vi "niRFUtil FTW Apply Window (complex wfm).vi"(3 "Window":T1=enum."Gaussian", 5 "Waveform In":T2 {"y" format="%.2f"; "dx" format="%^.2e"; "x0" format="%^.2e"}) -> (0 "-ENBW (dB-Hz)":sgl format="%.2f", 1 "Coherent Loss (dB)":sgl format="%.2f", 2 "Waveform Out":T2 {"y" format="%.2f"; "dx" format="%^.2e"; "x0" format="%^.2e"})   [LabVIEW 2015, in "niRFUtil.lvlib"]
doc: "(c) Copyright 2006, National Instruments, Inc. This VI may not be duplicated, sold, or distributed without written consent from National Instruments."
uses:
  niRFUtil.lvlib
  Includes/niRFUtil INC Complex Waveform.ctl
  Includes/niRFUtil INC Complex Array.ctl
  Includes/niRFUtil INC FFT Window.ctl
  <vilib>/Analysis/4window.llb/Hanning Window (CDB).vi
  <vilib>/Analysis/4window.llb/Hamming Window (CDB).vi
  <vilib>/Analysis/4window.llb/Gaussian Window (CDB).vi
  <vilib>/Analysis/4window.llb/Blackman Window (CDB).vi
  <vilib>/Analysis/4window.llb/Blackman-Harris Window (CDB).vi
  <vilib>/Analysis/4window.llb/Kaiser-Bessel Window (CDB).vi
  <vilib>/Analysis/4window.llb/AllCosWindow (CDB).vi
  <vilib>/Analysis/NI_AALPro.lvlib
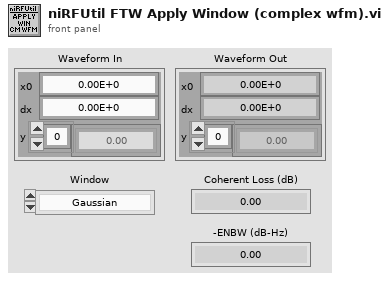
[diagram p1: front panel]
types:
  T1 = typedef "niRFUtil.lvlib/niRFUtil INC FFT Window.ctl" = enum16{"None", "Flat Top", "Hanning", "Hamming", "Gaussian", "Blackman", "Blackman-Harris", "Kaiser-Bessel 70 dB", "Kaiser-Bessel 90 dB", "Kaiser-Bessel 110 dB"}
  T2 = typedef "niRFUtil.lvlib/niRFUtil INC Complex Waveform.ctl" = cluster{"x0":dbl, "dx":dbl, "y":T3}
  T3 = typedef "niRFUtil.lvlib/niRFUtil INC Complex Array.ctl" = csg[]
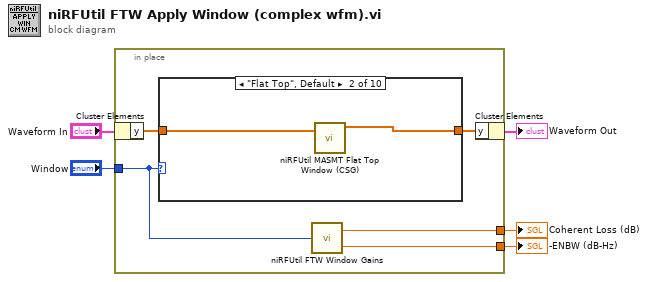
[diagram p0: block diagram]
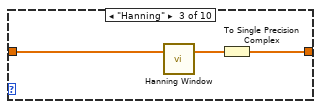
[diagram p3: hidden frame]
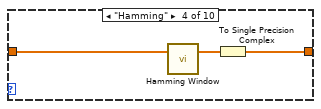
[diagram p4: hidden frame]
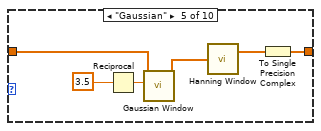
[diagram p5: hidden frame]
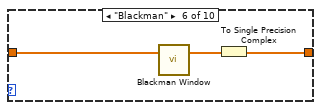
[diagram p6: hidden frame]
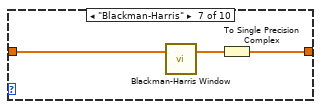
[diagram p7: hidden frame]
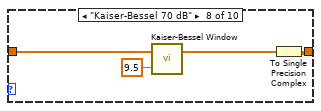
[diagram p8: hidden frame]
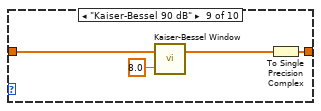
[diagram p9: hidden frame]
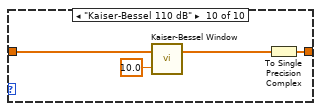
[diagram p10: hidden frame]
diagram:
  n1 = in-place {
    in-place-border: "Window" -> [w10]
    in-place-border: [w9] -> w4
    in-place-border: [w8] -> w3
    n2 = in-place-cluster #1("Waveform In") -> ("y"=w7:T3)
    n3 = case shown="\"Flat Top\", Default" w10 {
      tunnel: w7 -> [w11 w13 w16 w19 w25 w28 w31 w35 w39 w43]
      tunnel: [w11 w12 w14 w17 w20 w26 w29 w33 w37 w41] -> w6
      frame "None" {
      }
      frame "Flat Top", Default {
        n4 = call "niRFUtil MASMT Flat Top Window (CSG).vi"("X"=w13) -> ("Windowed X"=w12:csg[])  [unwired: 9 in, 1 out]
      }
      frame "Hanning" {
        n5 = call-poly <vilib>:"Hanning Window.vi"("X"=w16) -> ("Windowed X"=w15:cdb[])  [unwired: 1 out]
        n6 = To Single Precision Complex(1:w15) -> (0:w14:csg[])
      }
      frame "Hamming" {
        n7 = call-poly <vilib>:"Hamming Window.vi"("X"=w19) -> ("Windowed X"=w18:cdb[])  [unwired: 1 out]
        n8 = To Single Precision Complex(1:w18) -> (0:w17:csg[])
      }
      frame "Gaussian" {
        n9 = Reciprocal(x=3.5 ("standard deviation")) -> (1/x=w23:dbl)
        n10 = call-poly <vilib>:"Gaussian Window.vi"("standard deviation"=w23, "X"=w25) -> ("Windowed X"=w22:cdb[])  [unwired: 9 out]
        n11 = call-poly <vilib>:"Hanning Window.vi"("X"=w22) -> ("Windowed X"=w21:cdb[])  [unwired: 1 out]
        n12 = To Single Precision Complex(1:w21) -> (0:w20:csg[])
      }
      frame "Blackman" {
        n13 = call-poly <vilib>:"Blackman Window.vi"("X"=w28) -> ("Windowed X"=w27:cdb[])  [unwired: 1 out]
        n14 = To Single Precision Complex(1:w27) -> (0:w26:csg[])
      }
      frame "Blackman-Harris" {
        n15 = call-poly <vilib>:"Blackman-Harris Window.vi"("X"=w31) -> ("Windowed X"=w30:cdb[])  [unwired: 1 out]
        n16 = To Single Precision Complex(1:w30) -> (0:w29:csg[])
      }
      frame "Kaiser-Bessel 70 dB" {
        n17 = call-poly <vilib>:"Kaiser-Bessel Window.vi"("beta"=9.5, "X"=w35) -> ("Windowed X"=w32:cdb[])  [unwired: 1 out]
        n18 = To Single Precision Complex(1:w32) -> (0:w33:csg[])
      }
      frame "Kaiser-Bessel 90 dB" {
        n19 = call-poly <vilib>:"Kaiser-Bessel Window.vi"("beta"=8.0, "X"=w39) -> ("Windowed X"=w36:cdb[])  [unwired: 1 out]
        n20 = To Single Precision Complex(1:w36) -> (0:w37:csg[])
      }
      frame "Kaiser-Bessel 110 dB" {
        n21 = call-poly <vilib>:"Kaiser-Bessel Window.vi"("beta"=10.0, "X"=w43) -> ("Windowed X"=w40:cdb[])  [unwired: 1 out]
        n22 = To Single Precision Complex(1:w40) -> (0:w41:csg[])
      }
    }
    n23 = call "niRFUtil FTW Window Gains.vi"("Window"=w10) -> ("-ENBW (dB-Hz)"=w8:sgl, "Coherent Loss (dB)"=w9:sgl)  [unwired: 2 in]
    n24 = in-place-cluster #1("y"=w6) -> (→"Waveform Out":T2)
  }
  "-ENBW (dB-Hz)" <- w3
  "Coherent Loss (dB)" <- w4
